vi "Write Active Plot.vi"(8 "error in (no error)":errorcluster, 10 "Active Plot":i32, 11 "2D Feather.lvclass in":refnum<class "2D Feather.lvclass">) -> (0 "error out":errorcluster, 3 "2D Feather.lvclass out":refnum<class "2D Feather.lvclass">)   [LabVIEW 2020, in "2D Feather.lvclass"]
uses:
  <vilib>/Math Plots/2D Math Plots/2D Feather/2D Feather/2D Feather.lvclass
  <vilib>/Math Plots/2D Math Plots/2D Feather/2D Feather/2D Feather.lvclass/2D Feather.ctl
  <vilib>/Math Plots/2D Math Plots/2D Feather/2D Feather/Typedef/2D Feather Property.ctl
  <vilib>/Math Plots/2D Math Plots/2D Plot/2D Plot/2D Plot.lvclass
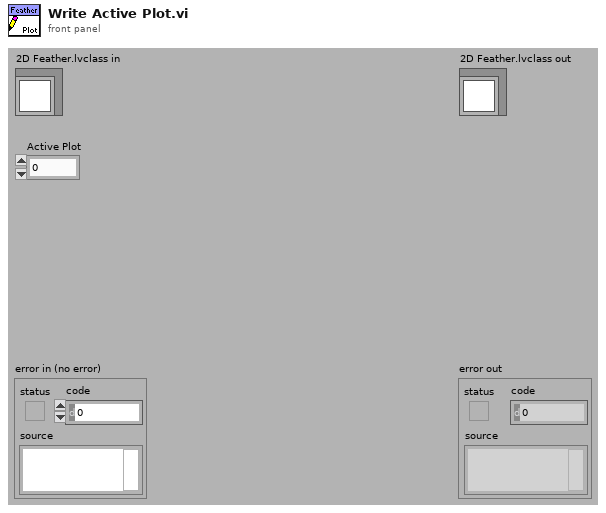
[diagram p1: front panel]
types:
  T1 = typedef "2D Feather.lvclass/2D Feather Property.ctl" = cluster{"Arrow Size":dbl}
  T2 = typedef "2D Plot.lvclass/Plot Property Array.ctl" = T3[]
  T3 = typedef "2D Plot.lvclass/Plot Property.ctl" = cluster{"Bar Plot Style":u8, "DigitalLineStyle":u8, "TransitionLocation":u8, "Transition Type":u8, "Fill To":i16, "Fill/Pt. Color":u32, "Label Style":u8, "Line Style":u8, "Line Width":u8, "Plot Color":u32, "Plot Interpolation":u8, "Plot Name":string, "Point Style":u8, "Visible?":bool, "XScaleIdx":u32, "YScaleIdx":u32}
  T4 = typedef "2D Feather.lvclass/2D Feather Property Array.ctl" = T1[]
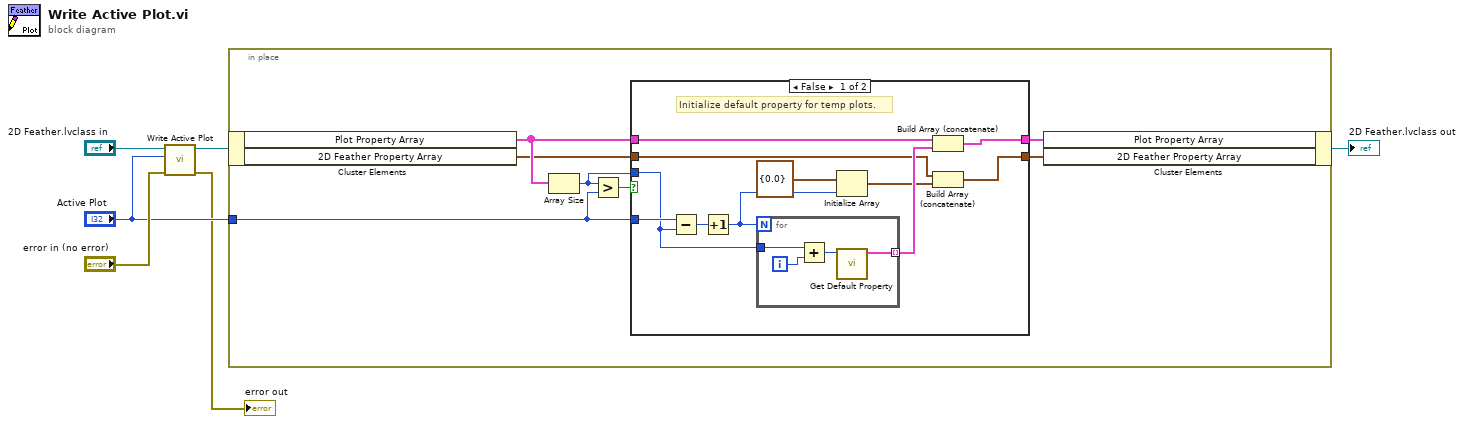
[diagram p0: block diagram]
diagram:
  n1 = call-parent "Write Active Plot.vi"("error in (no error)"="error in (no error)", "Active Plot"="Active Plot", "2D Plot.lvclass in"="2D Feather.lvclass in") -> ("error out"=→"error out":errorcluster, "2D Plot.lvclass out"=w4:refnum<class "2D Feather.lvclass">)  [unwired: 7 in]
  n2 = in-place {
    in-place-border: "Active Plot" -> [w11]
    n3 = in-place-cluster #1(w4) -> ("Plot Property Array"=w12:T2, "2D Feather Property Array"=w8:T4)
    n4 = Array Size(array=w12) -> (size(s)=w10:i32)
    n5 = Greater?(x=w10, y=w11) -> (0:w13:bool)
    n6 = case shown="False" w13 {
      tunnel: [w22 w30] -> w9
      tunnel: w12 -> [w24 w30]
      tunnel: w10 -> [w19 _]
      tunnel: w11 -> [w20 _]
      tunnel: w8 -> [w18 w29]
      tunnel: [w17 w29] -> w7
      frame False {
        # "Initialize default property for temp plots."
        n7 = Subtract(x=w20, y=w19) -> (x-y=w21:i32)
        n8 = Increment(x=w21) -> (x+1=w16:i32)
        n9 = for {
          N: w16 -> [_]
          tunnel: w19 -> [w27]
          tunnel: [w26] -> w23 mode=indexing
          i -> [w28]
          n10 = Add(x=w27, y=w28) -> (x+y=w25:i32)
          n11 = call <vilib>:"Get Default Property.vi"("Index"=w25) -> ("Temporary Property"=w26:T3)  [unwired: 10 in]
        }
        n12 = Initialize Array(T1 {"Arrow Size"=0.0} ("2D Feather Property"), w16) -> (w15:T1[])
        n13 = Build Array (concatenate)(w24, w23) -> (w22:T2)
        n14 = Build Array (concatenate)(w18, w15) -> (w17:T4)
      }
      frame True {
      }
    }
    n15 = in-place-cluster #1("Plot Property Array"=w9, "2D Feather Property Array"=w7) -> (→"2D Feather.lvclass out":refnum<class "2D Feather.lvclass">)
  }
